vi "Update Display.vi"(8 "Error In":errorcluster, 9 "string":string, 10 "Action":enum16{"Add String", "Newline", "Clear"}(ring), 11 "Display In":refnum<vi>) -> (0 "Error Out":errorcluster, 3 "Display Out":refnum<vi>)   [LabVIEW 2014]
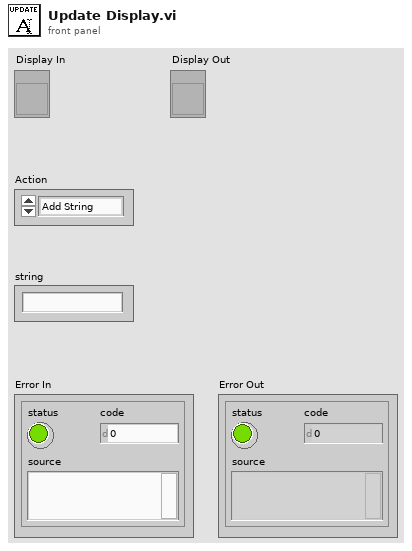
[diagram p1: front panel]
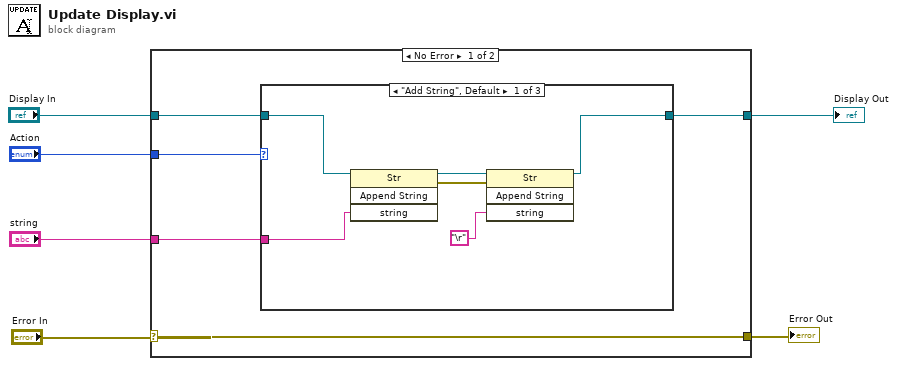
[diagram p0: block diagram]
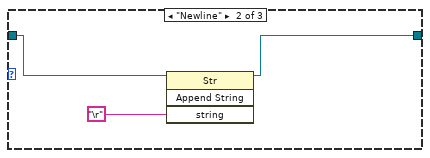
[diagram p2: hidden frame]
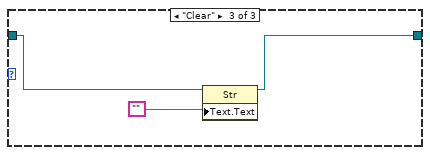
[diagram p3: hidden frame]
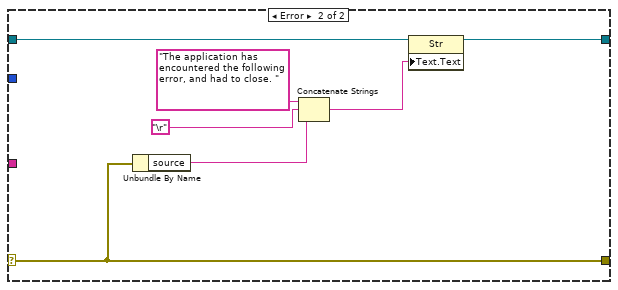
[diagram p4: hidden frame]
diagram:
  n1 = case shown="No Error" "Error In" {
    selector: "Error In" -> [w7 w24]
    tunnel: "Display In" -> [w11 w30]
    tunnel: "Action" -> [w10 _]
    tunnel: [w9 w29] -> w4
    tunnel: "string" -> [w8 _]
    tunnel: [w7 w24] -> w1
    frame No Error {
      n2 = case shown="\"Add String\", Default" w10 {
        tunnel: w11 -> [w17 w19 w23]
        tunnel: [w14 w18 w22] -> w9
        tunnel: w8 -> [w13 _ _]
        frame "Add String", Default {
          n3 = invoke class="Str" method="Append String"(reference=w17, "string"=w13) -> (reference out=w16:refnum<vi>, error out=w15:errorcluster)  [unwired: 2 in, 2 out]
          n4 = invoke class="Str" method="Append String"(reference=w16, error in=w15, "string"="\r") -> (reference out=w14:refnum<vi>)  [unwired: 1 in, 3 out]
        }
        frame "Newline" {
          n5 = invoke class="Str" method="Append String"(reference=w19, "string"="\r") -> (reference out=w18:refnum<vi>)  [unwired: 2 in, 3 out]
        }
        frame "Clear" {
          n6 = property class="Str"(reference=w23, "Text.Text"="") -> (reference out=w22:refnum<vi>)  [unwired: 1 in, 1 out]
        }
      }
    }
    frame Error {
      n7 = Unbundle By Name(w24) -> ("source"=w26:string)
      n8 = Concatenate Strings("The application has encountered the following error, and had to close. " ("string"), "\r", w26) -> (w25:string)
      n9 = property class="Str"(reference=w30, "Text.Text"=w25) -> (reference out=w29:refnum<vi>)  [unwired: 1 in, 1 out]
    }
  }
  "Display Out" <- w4
  "Error Out" <- w1
